vi "SJ_old_results plotter.vi"() -> ()   [LabVIEW 2022 SP3]
uses:
  Controls/Inst_type.ctl
  Controls/Instrument_Array.ctl
  Controls/Analysis_info_cluster.ctl
  Controls/SJ_Test_Matrix.ctl
  <vilib>/Analysis/NI_AALBase.lvlib
  <vilib>/Analysis/1siggen.llb/Ramp Pattern by Samples.vi
  <vilib>/Analysis/baseanly.llb/Scale 1D.vi
  <vilib>/Analysis/NI_AALPro.lvlib
  <vilib>/Analysis/baseanly.llb/Scale 2D.vi
  <vilib>/gmath/NumericalOptimization/stopping criteria.ctl
  <vilib>/gmath/NI_Gmath.lvlib
panel:
  out "size(s)":i32[](array[numeric])
  out "Tab Control":enum32{"Animate", "Parabola"}(tab)
  out "Displacement Graph":cluster{"Y=(X-offset)/scale":dbl[], dbl[]}[](graph)
  out "Progress...":sgl(slide) scale=0.0..1.0
  out "Error":cluster{dbl[], dbl[]}[](graph)
  out "Phi":cluster{dbl[], dbl[]}[](graph)
  out "Beta":cluster{dbl[], dbl[]}[](graph)
  in  "stopping criteria":T1={"function tolerance"=0.001, "parameter tolerance"=0.001, "max iterations"=100, "max function calls"=1000, "gradient tolerance"=0.001, "max time (sec)"=-1.0}
  in  "Fit Parabola":bool
  in  "Load data":bool
  in  "Raw Data Folder":path=path "F:/Enflo_Data_Local/2011/Aero_Tunnel/nick_martin/Raw_Measurements/11-2011/New_SJ_TestI_xls"
  in  "Play Button":bool
  out "Message":string
  in  "Frequencies":i32[](listbox)
  in  "Amplitudes":i32[](listbox)
  in  "Stop Button":bool
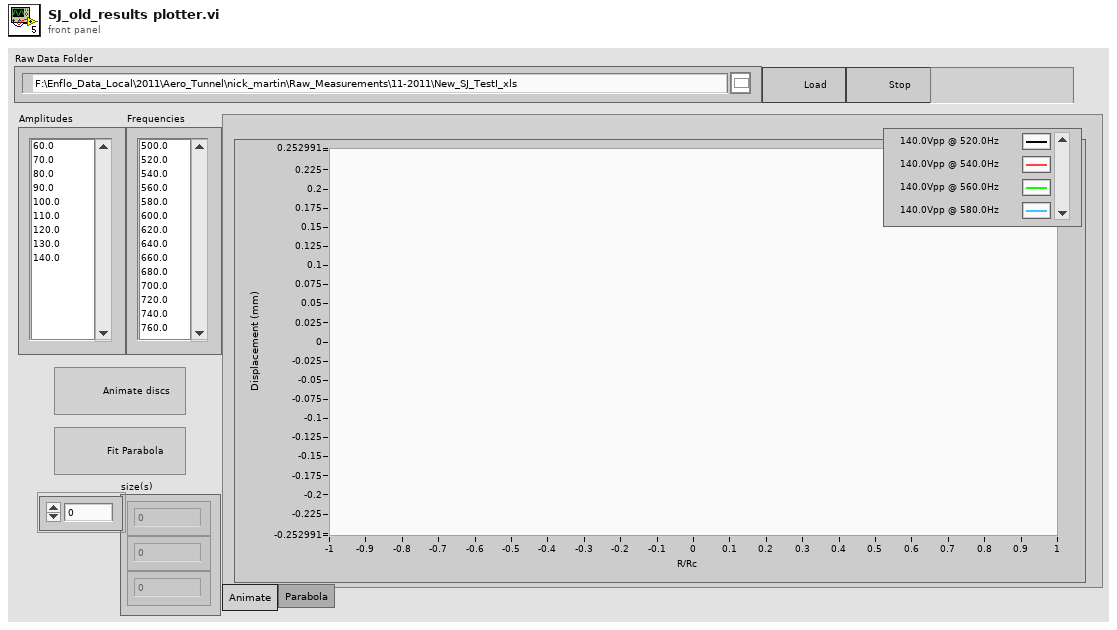
[diagram p1: front panel]
types:
  T1 = typedef "NI_Gmath.lvlib/stopping criteria.ctl" = cluster{"function tolerance":dbl, "parameter tolerance":dbl, "max iterations":i32, "max function calls":i32, "gradient tolerance":dbl, "max time (sec)":dbl}
  T2 = typedef "SJ_Test_Matrix.ctl" = cluster{"Channel Data":cluster{"Amplitude (V)":dbl, "Phase Average":dbl[][], "Phase Angle":dbl[], "Frequency (Hz)":dbl, "AS Freq":dbl, "Zero":dbl, "Analysis info cluster":T3, "Radius":dbl[], "||beta||":dbl, "Phi":dbl, "||xd'||":dbl, "xd":dbl[], "||xd||":dbl, "xd'":dbl[], "beta":dbl[]}[]}
  T3 = typedef "Analysis_info_cluster.ctl" = cluster{"Colour":u32, "Inst type":T4, "Inst name":string, "Symbol":string, "Code name":string, "Extra Info":string, "Inst Array":T5, "Extra Titles":string[], "Extra Values":string[], "U":dbl, "u^2":dbl, "u^3":dbl, "u^4":dbl, "Skew_u":dbl, "Kurt_u":dbl, "Sd Error in Mean":dbl, "% u'/U":dbl, "X":dbl, "Y":dbl, "Z":dbl, "Timescale integral Estimate":dbl, "Sd Error in Variance":dbl, "Calib File":path, "Calib Constants":dbl[], "Output Position":bool, "Stats":enum16{"None", "Basic", "Full"}, "Av Sampling Rate":dbl, "Av No of Samples":dbl, "Total Meas Time (s)":dbl, "ADAM Ch Name":string, "Max value":dbl, "Min value":dbl, "Req Sample Rate Hz":dbl, "Sync Delay Time (s)":dbl, "Ch No":i16, "Device":string, "Use Latest Calib":bool, "Port":string, "Metadata Ch Names":string[], "Metadata Ch Values":string[], "Label":string}
  T4 = typedef "Inst_type.ctl" = enum16{"Raw voltage", "Raw with zero offsetting", "Propeller anemometer", "Pressure Transducer", "Pitot-static tube", "Hot wire", "Cross wire 1", "Cross wire 2", "Generic Linear", "Generic Polynomial", "Generic BackPoly", "Fast FID", "Thermocouple", "Cold wire", "Pulsed Wire", "LDA Vel", "LDA Tran time", "LDA Arr time", "Microphone"}
  T5 = typedef "Instrument_Array.ctl" = enum16{"PWA", "LDA", "Analogue"}
  T6 = cluster{"Amplitude (V)":dbl, "Phase Average":dbl[][], "Phase Angle":dbl[], "Frequency (Hz)":dbl, "AS Freq":dbl, "Zero":dbl, "Analysis info cluster":T3, "Radius":dbl[], "||beta||":dbl, "Phi":dbl, "||xd'||":dbl, "xd":dbl[], "||xd||":dbl, "xd'":dbl[], "beta":dbl[]}[]
  T7 = cluster{"Amplitude (V)":dbl, "Phase Average":dbl[][], "Phase Angle":dbl[], "Frequency (Hz)":dbl, "AS Freq":dbl, "Zero":dbl, "Analysis info cluster":T3, "Radius":dbl[], "||beta||":dbl, "Phi":dbl, "||xd'||":dbl, "xd":dbl[], "||xd||":dbl, "xd'":dbl[], "beta":dbl[]}
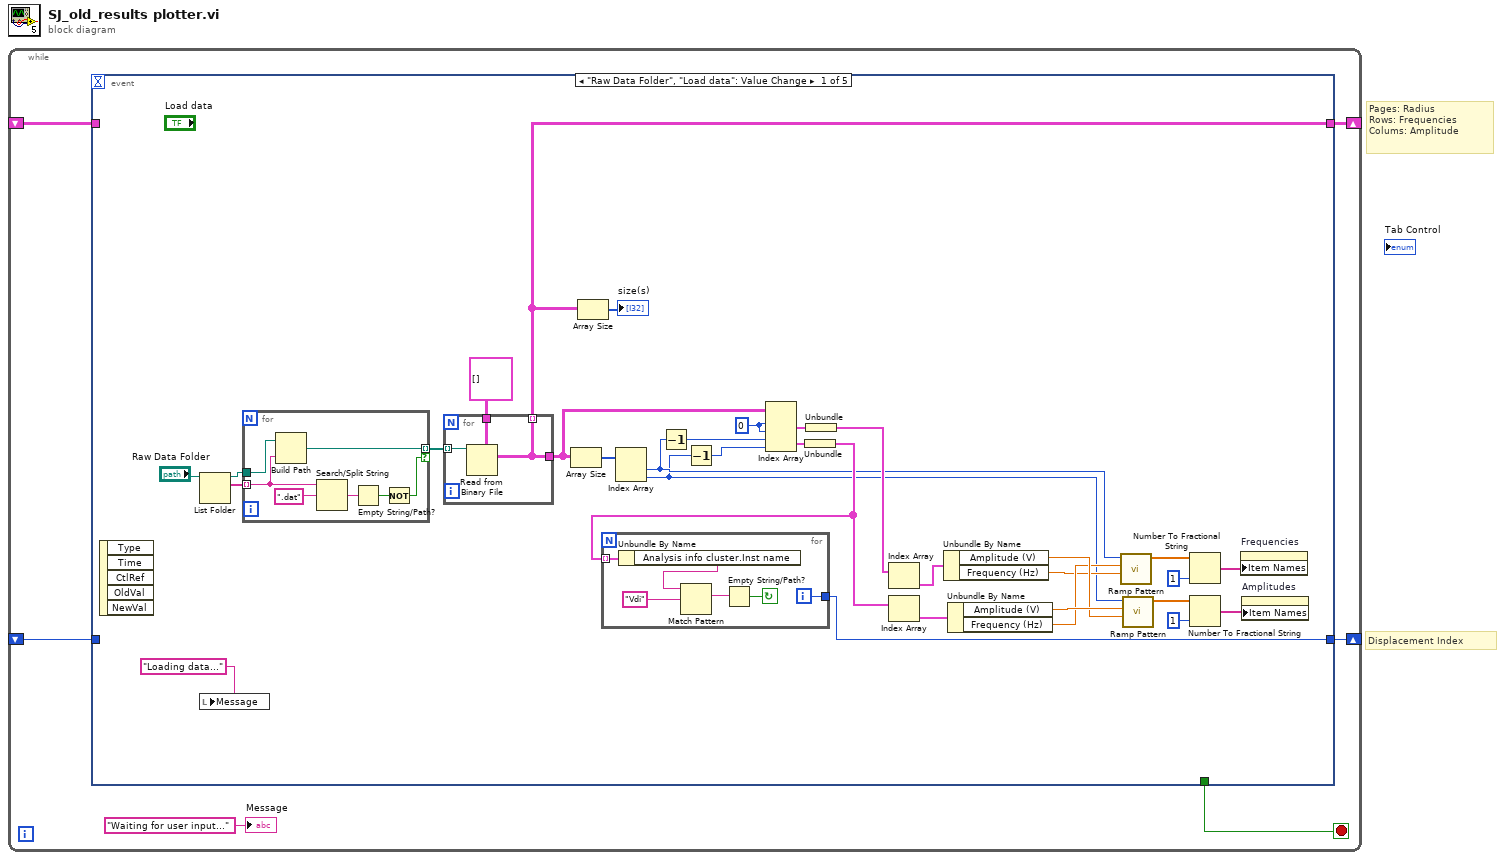
[diagram p0: block diagram]
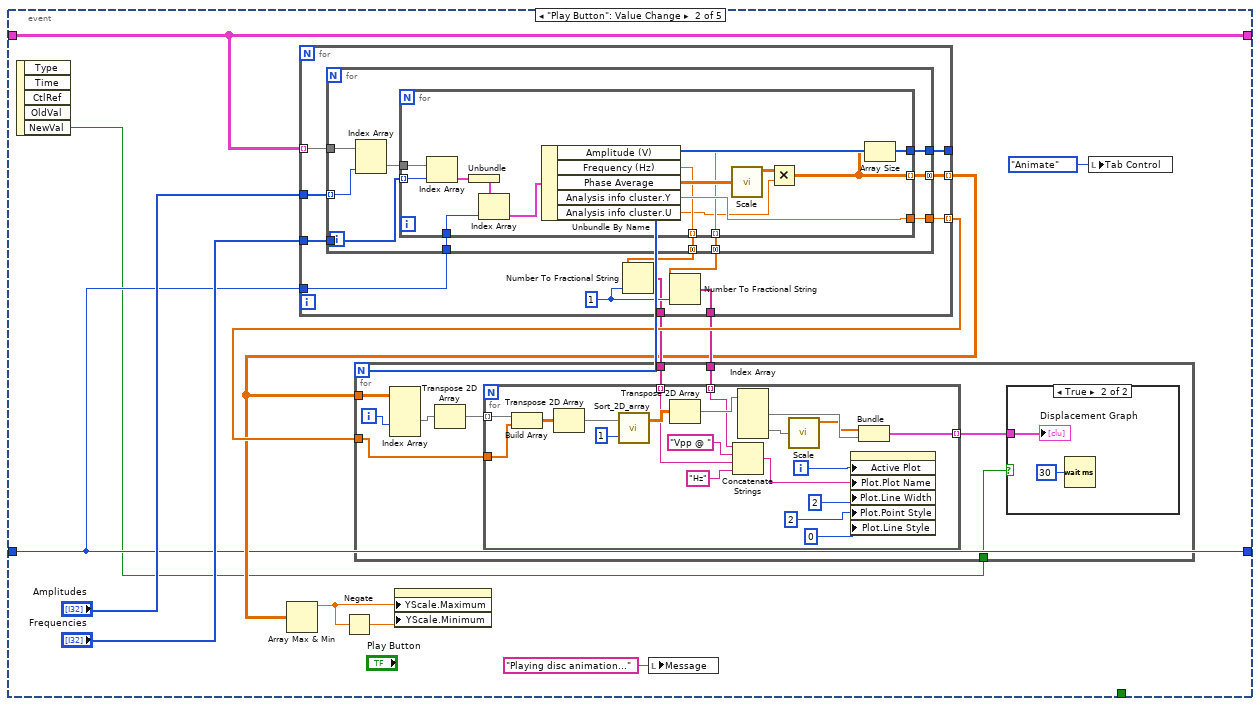
[diagram p2: hidden frame]
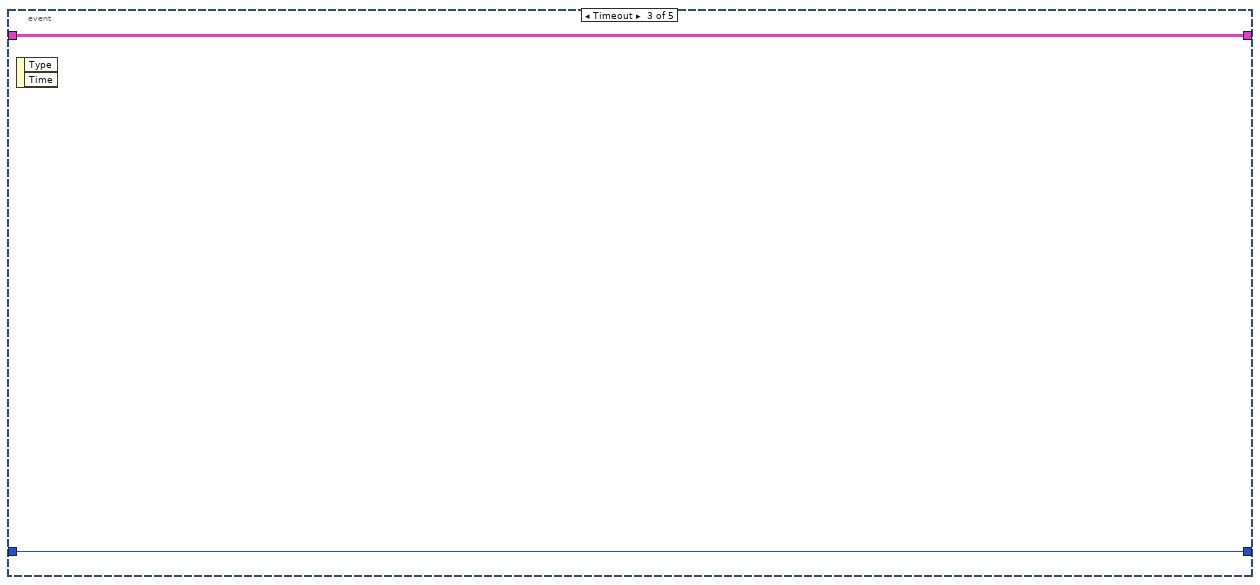
[diagram p4: hidden frame]
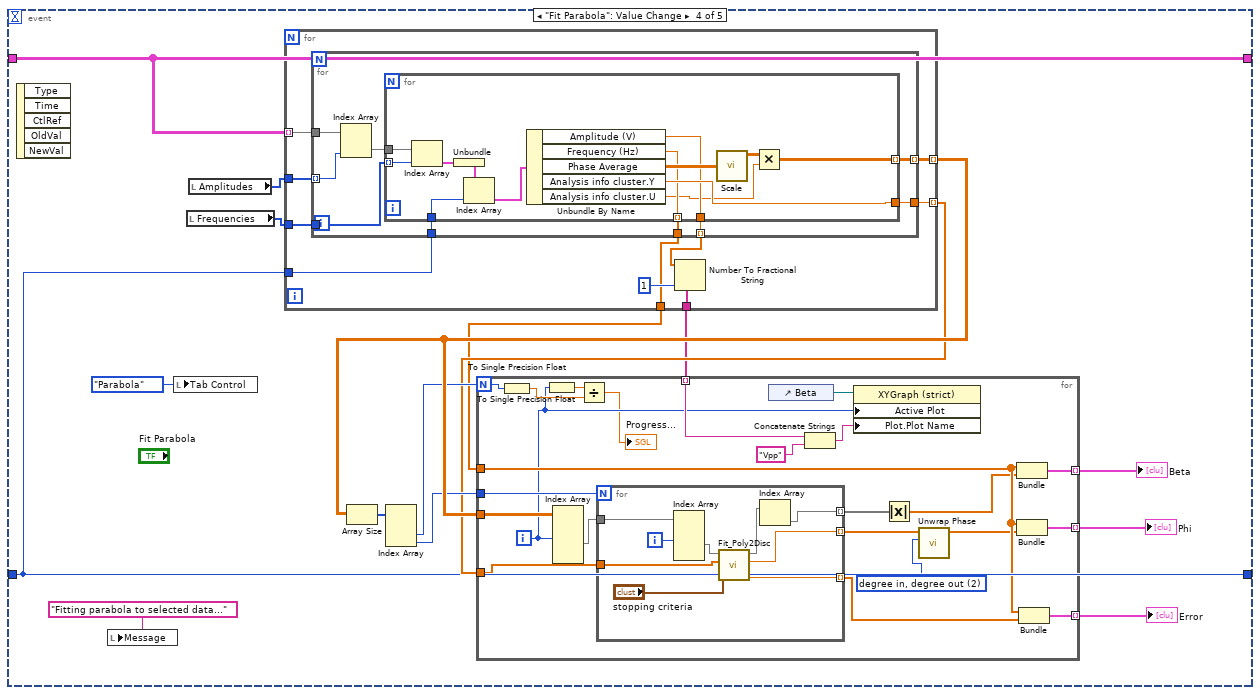
[diagram p5: hidden frame]
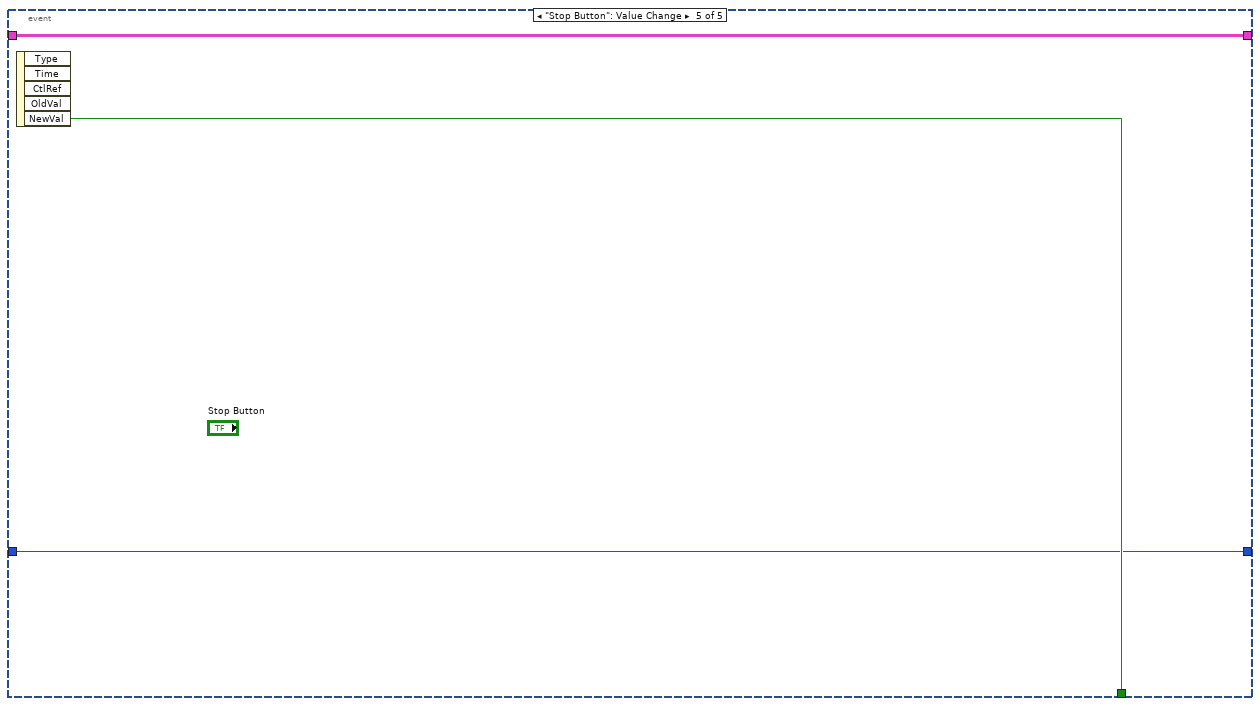
[diagram p6: hidden frame]
diagram:
  # "Displacement Index"
  # "Pages: Radius\nRows: Frequencies\nColums: Amplitude"
  n1 = while {
    shift-right: [w2] -> _
    shift-left: _ -> [w5]
    shift-right: [w3] -> _
    shift-left: _ -> [w4]
    stop <- w6 stop-if-true
    n2 = event shown="[0] \"Raw Data Folder\", \"Load data\": Value Change" {
      selector: _ -> [_ _ _ _ _]
      dyn-events: _ -> [_ _ _ _ _]
      timeout: _ -> [_ _ _ _ _]
      tunnel: [_ _ _ _ w220] -> w6
      tunnel: w5 -> [_ w65 w136 w138 w219]
      tunnel: w4 -> [_ w57 w137 w142 w218]
      tunnel: [w10 w57 w137 w142 w218] -> w3
      tunnel: [w8 w65 w136 w138 w219] -> w2
      event "Raw Data Folder", "Load data": Value Change {
        w17 = 0 ("index (row)")
        n3 = event-data() -> ()  [unwired: 1 in, 5 out]
        n4 = List Folder(path="Raw Data Folder") -> (path out=w36:path, filenames=w37:string[])  [unwired: 3 in, 2 out]
        n5 = local write "Message"("Loading data..." ("Message")) -> ()
        n6 = for {
          tunnel: w37 -> [w49] mode=indexing
          tunnel: [w48] -> w23 mode=indexing if=w52
          tunnel: w36 -> [w50]
          n7 = Build Path(base path=w50, name or relative path=w49) -> (appended path=w48:path)
          n8 = Search/Split String(string=w49, search string/char (-)=".dat" ("regular expression")) -> (match + rest of string=w51:string)  [unwired: 1 in, 2 out]
          n9 = Empty String/Path?(string/path=w51) -> (empty?=w53:bool)
          n10 = Not(x=w53) -> (.not. x?=w52:bool)
        }
        n11 = for {
          tunnel: w23 -> [w47] mode=indexing
          tunnel: T2[][] [] -> [w46]
          tunnel: [w45] -> w15
          tunnel: [w45] -> w8 mode=indexing
          n12 = Read from Binary File(5:w46, 11:w47) -> (2:w45:T2[][])  [unwired: 4 in, 3 out]
        }
        n13 = Array Size(array=w15) -> (size(s)=w16:i32[])
        n14 = Array Size(array=w8) -> (size(s)=→"size(s)":i32[])
        n15 = Index Array(array=w16) -> (element #1=w12:i32, element #2=w11:i32)  [unwired: 2 in]
        n16 = Decrement(x=w12) -> (x-1=w18:i32)
        n17 = Decrement(x=w11) -> (x-1=w19:i32)
        n18 = Index Array(array=w15, index (row) #1=w17, index (col) #1=w17, index (row) #2=w18, index (col) #2=w19) -> (element #1=w20:T2, element #2=w21:T2)
        n19 = Unbundle(w21) -> ("Channel Data"=w14:T6)
        n20 = for {
          tunnel: w14 -> [w44] mode=indexing
          tunnel: [w39] -> w10
          i -> [w39]
          stop <- w40 continue-if-true
          n21 = Unbundle By Name(w44) -> ("Analysis info cluster.Inst name"=w43:string)
          n22 = Match Pattern(string=w43, regular expression="Vdi") -> (match substring=w41:string)  [unwired: 1 in, 3 out]
          n23 = Empty String/Path?(string/path=w41) -> (empty?=w40:bool)
        }
        n24 = Unbundle(w20) -> ("Channel Data"=w13:T6)
        n25 = Index Array(array=w13) -> (element=w31:T7)  [unwired: 1 in]
        n26 = Index Array(array=w14) -> (element=w32:T7)  [unwired: 1 in]
        n27 = Unbundle By Name(w31) -> ("Amplitude (V)"=w34:dbl, "Frequency (Hz)"=w30:dbl)
        n28 = Unbundle By Name(w32) -> ("Amplitude (V)"=w35:dbl, "Frequency (Hz)"=w33:dbl)
        n29 = call-poly <vilib>:"Ramp Pattern.vi"("start"=w30, "end"=w33, "samples"=w12) -> ("Ramp Pattern"=w29:dbl[])  [unwired: 7 in, 1 out]
        n30 = call-poly <vilib>:"Ramp Pattern.vi"("start"=w34, "end"=w35, "samples"=w11) -> ("Ramp Pattern"=w27:dbl[])  [unwired: 7 in, 1 out]
        n31 = Number To Fractional String(number=w29, precision (6)=i16 1) -> (F-format string=w28:string[])  [unwired: 2 in]
        n32 = Number To Fractional String(number=w27, precision (6)=i16 1) -> (F-format string=w26:string[])  [unwired: 2 in]
        n33 = property on="Frequencies" class="LstBox (strict)"("Item Names"=w28) -> ()  [unwired: 2 in, 2 out]
        n34 = property on="Amplitudes" class="LstBox (strict)"("Item Names"=w26) -> ()  [unwired: 2 in, 2 out]
      }
      event "Play Button": Value Change {
        n35 = event-data() -> ("NewVal"=w56:bool)  [unwired: 1 in, 4 out]
        n36 = for {
          tunnel: w65 -> [w111] mode=indexing
          tunnel: [w110] -> w66 mode=indexing
          tunnel: "Amplitudes" -> [w109]
          tunnel: "Frequencies" -> [w108]
          tunnel: [w107] -> w60 mode=indexing
          tunnel: [w106] -> w67
          tunnel: [w104] -> w64
          tunnel: [w101] -> w63
          tunnel: w57 -> [w100]
          w102 = i16 1 ("precision (6)")
          n37 = for {
            tunnel: w111 -> [w121]
            tunnel: [w119] -> w110
            tunnel: [w118] -> w107 mode=concatenating
            tunnel: w109 -> [w117] mode=indexing
            tunnel: w108 -> [w116]
            tunnel: [w115] -> w106
            tunnel: [w114] -> w103 mode=concatenating
            tunnel: [w113] -> w105 mode=concatenating
            tunnel: w100 -> [w112]
            n38 = Index Array(array=w121, index (col)=w117) -> (element=w120:T2[])  [unwired: 1 in]
            n39 = for {
              tunnel: w120 -> [w135]
              tunnel: [w131] -> w119
              tunnel: [w123] -> w118 mode=indexing
              tunnel: w116 -> [w128] mode=indexing
              tunnel: [w127] -> w115
              tunnel: [w126] -> w114 mode=indexing
              tunnel: [w125] -> w113 mode=indexing
              tunnel: w112 -> [w122]
              n40 = Index Array(array=w135, index=w128) -> (element=w134:T2)
              n41 = Unbundle(w134) -> ("Channel Data"=w133:T6)
              n42 = Index Array(array=w133, index=w122) -> (element=w132:T7)
              n43 = Unbundle By Name(w132) -> ("Amplitude (V)"=w125:dbl, "Frequency (Hz)"=w126:dbl, "Phase Average"=w130:dbl[][], "Analysis info cluster.Y"=w131:dbl, "Analysis info cluster.U"=w124:dbl)
              n44 = call-poly <vilib>:"Scale.vi"("X"=w130) -> ("Y=(X-offset)/scale"=w129:dbl[][])  [unwired: 3 out]
              n45 = Multiply(x=w129, y=w124) -> (x*y=w123:dbl[][])
              n46 = Array Size(array=w123) -> (size(s)=w127:i32[])
            }
          }
          n47 = Number To Fractional String(number=w103, precision (6)=w102) -> (F-format string=w101:string[])  [unwired: 2 in]
          n48 = Number To Fractional String(number=w105, precision (6)=w102) -> (F-format string=w104:string[])  [unwired: 2 in]
        }
        n49 = Array Max & Min(array=w60) -> (max value=w62:dbl)  [unwired: 3 out]
        n50 = Negate(x=w62) -> (-x=w61:dbl)
        n51 = for {
          N: w67 -> [_]
          tunnel: w66 -> [w77]
          tunnel: w60 -> [w72]
          tunnel: w56 -> [w75]
          tunnel: w64 -> [w74]
          tunnel: w63 -> [w73]
          i -> [w69]
          n52 = Index Array(array=w72, index (dim 2)=w69) -> (element=w70:dbl[][][])  [unwired: 3 in]
          n53 = Transpose 2D Array(2D array=w70) -> (transposed array=w71:dbl[][])
          n54 = for {
            tunnel: w71 -> [w99] mode=indexing
            tunnel: w77 -> [w87]
            tunnel: [w84] -> w76 mode=indexing
            tunnel: w74 -> [w92] mode=indexing
            tunnel: w73 -> [w90] mode=indexing
            i -> [w82]
            n55 = Build Array(w99, w87) -> (w98:dbl[][])
            n56 = Transpose 2D Array(2D array=w98) -> (transposed array=w94:dbl[][])
            n57 = call "Sort_2D_array.vi"("Column index to sort on"=1, "unsorted array"=w94) -> ("sorted array"=w96:dbl[][])  [unwired: 1 out]
            n58 = Transpose 2D Array(2D array=w96) -> (transposed array=w93:dbl[][])
            n59 = Concatenate Strings(w92, "Vpp @ " ("string"), w90, "Hz" ("string")) -> (w88:string)
            n60 = Index Array(array=w93) -> (element #1=w95:dbl[], element #2=w86:dbl[])  [unwired: 4 in]
            n61 = call-poly <vilib>:"Scale.vi"("X"=w86) -> ("Y=(X-offset)/scale"=w85:dbl[])  [unwired: 3 out]
            n62 = property on="Displacement Graph" class="XYGraph (strict)"("Active Plot"=w82, "Plot.Plot Name"=w88, "Plot.Line Width"=u8 2, "Plot.Point Style"=u8 2, "Plot.Line Style"=u8 0) -> ()  [unwired: 2 in, 2 out]
            n63 = Bundle("Y=(X-offset)/scale"=w85, w95) -> (w84:cluster{"Y=(X-offset)/scale":dbl[], dbl[]})  [unwired: 1 in]
          }
          n64 = case shown="True" w75 {
            tunnel: w76 -> [_ w78]
            frame False {
            }
            frame True {
              n65 = Wait (ms)(milliseconds to wait=u32 30) -> ()  [unwired: 1 out]
              "Displacement Graph" <- w78
            }
          }
        }
        n66 = property on="Displacement Graph" class="XYGraph (strict)"("YScale.Maximum"=w62, "YScale.Minimum"=w61) -> ()  [unwired: 2 in, 2 out]
        n67 = local write "Message"("Playing disc animation..." ("Message")) -> ()
        n68 = local write "Tab Control"(enum32{"Animate", "Parabola"}."Animate" ("Tab Control")) -> ()
      }
      event Timeout {
        n69 = event-data() -> ()  [unwired: 1 in, 2 out]
      }
      event "Fit Parabola": Value Change {
        n70 = event-data() -> ()  [unwired: 1 in, 5 out]
        n71 = local write "Message"("Fitting parabola to selected data..." ("Message")) -> ()
        n72 = local write "Tab Control"(enum32{"Animate", "Parabola"}."Parabola" ("Tab Control")) -> ()
        n73 = local read "Frequencies"() -> (w143:i32[])
        n74 = local read "Amplitudes"() -> (w144:i32[])
        n75 = for {
          tunnel: w138 -> [w195] mode=indexing
          tunnel: [w194] -> w148 mode=indexing
          tunnel: w144 -> [w193]
          tunnel: w143 -> [w192]
          tunnel: [w191] -> w152 mode=indexing
          tunnel: [w190] -> w145
          tunnel: w142 -> [w188]
          tunnel: [w186] -> w147
          n76 = for {
            tunnel: w195 -> [w204]
            tunnel: [w202] -> w194
            tunnel: [w201] -> w191 mode=indexing
            tunnel: w193 -> [w200] mode=indexing
            tunnel: w192 -> [w199]
            tunnel: [w198] -> w186
            tunnel: [w197] -> w187 mode=indexing
            tunnel: w188 -> [w196]
            n77 = Index Array(array=w204, index (col)=w200) -> (element=w203:T2[])  [unwired: 1 in]
            n78 = for {
              tunnel: w203 -> [w217]
              tunnel: [w213] -> w202
              tunnel: [w206] -> w201 mode=indexing
              tunnel: w199 -> [w210] mode=indexing
              tunnel: [w209] -> w198 mode=indexing
              tunnel: [w208] -> w197
              tunnel: w196 -> [w205]
              n79 = Index Array(array=w217, index=w210) -> (element=w216:T2)
              n80 = Unbundle(w216) -> ("Channel Data"=w215:T6)
              n81 = Index Array(array=w215, index=w205) -> (element=w214:T7)
              n82 = Unbundle By Name(w214) -> ("Amplitude (V)"=w208:dbl, "Frequency (Hz)"=w209:dbl, "Phase Average"=w212:dbl[][], "Analysis info cluster.Y"=w213:dbl, "Analysis info cluster.U"=w207:dbl)
              n83 = call-poly <vilib>:"Scale.vi"("X"=w212) -> ("Y=(X-offset)/scale"=w211:dbl[][])  [unwired: 3 out]
              n84 = Multiply(x=w211, y=w207) -> (x*y=w206:dbl[][])
            }
          }
          n85 = Number To Fractional String(number=w187, precision (6)=i16 1) -> (F-format string=w190:string[])  [unwired: 2 in]
        }
        n86 = Array Size(array=w152) -> (size(s)=w151:i32[])
        n87 = Index Array(array=w151) -> (element #2=w150:i32, element #3=w149:i32)  [unwired: 3 in, 1 out]
        n88 = for {
          N: w150 -> [w161]
          tunnel: w152 -> [w176]
          tunnel: w149 -> [w174]
          tunnel: w148 -> [w173]
          tunnel: w147 -> [w166]
          tunnel: [w169] -> w146 mode=indexing
          tunnel: [w168] -> w140 mode=indexing
          tunnel: [w167] -> w139 mode=indexing
          tunnel: w145 -> [w165] mode=indexing
          i -> [w158]
          w154 = 2 items=["radian in, radian out", "radian in, degree out", "degree in, degree out", "degree in, radian out"] ("phase unit")
          n89 = To Single Precision Float(number=w161) -> (single precision float=w160:sgl)
          n90 = To Single Precision Float(number=w158) -> (single precision float=w159:sgl)
          n91 = Index Array(array=w176, index (dim 1)=w158) -> (element=w175:dbl[][][][])  [unwired: 4 in]
          n92 = Divide(x=w159, y=w160) -> (x/y=→"Progress...":sgl)
          n93 = for {
            N: w174 -> [_]
            tunnel: w175 -> [w185]
            tunnel: w173 -> [w183]
            tunnel: [w181] -> w172 mode=indexing
            tunnel: [w180] -> w171 mode=indexing
            tunnel: [w179] -> w170 mode=indexing
            i -> [w184]
            n94 = Index Array(array=w185, index (dim 1)=w184) -> (element=w178:dbl[][][])  [unwired: 3 in]
            n95 = call "Fit_Poly2Disc.vi"("stopping criteria"="stopping criteria", "Rc"=w183, "Xd(t,r)"=w178) -> ("f(minimum)"=w179:dbl, "Sine Phase"=w180:dbl, 3:w182)  [unwired: 5 in, 1 out]
            n96 = Index Array(array=w182) -> (element=w181)  [unwired: 1 in]
          }
          n97 = control-ref of="Beta"() -> (w164:refnum<vi>)
          n98 = Concatenate Strings(w165, "Vpp" ("string")) -> (w163:string)
          n99 = property class="XYGraph (strict)"(reference=w164, "Active Plot"=w158, "Plot.Plot Name"=w163) -> ()  [unwired: 1 in, 2 out]
          n100 = Absolute Value(x=w172) -> (abs(x)=w156:dbl[])
          n101 = call <vilib>:"Unwrap Phase.vi"("phase unit"=w154, "Phase"=w171) -> ("Unwrapped Phase"=w155:dbl[])  [unwired: 8 in, 1 out]
          n102 = Bundle(w166, w156) -> (w169:cluster{dbl[], dbl[]})  [unwired: 1 in]
          n103 = Bundle(w166, "Unwrapped Phase"=w155) -> (w168:cluster{dbl[], "Unwrapped Phase":dbl[]})  [unwired: 1 in]
          n104 = Bundle(w166, w170) -> (w167:cluster{dbl[], dbl[]})  [unwired: 1 in]
        }
        "Beta" <- w146
        "Phi" <- w140
        "Error" <- w139
      }
      event "Stop Button": Value Change {
        n105 = event-data() -> ("NewVal"=w220:bool)  [unwired: 1 in, 4 out]
      }
    }
    "Message" <- "Waiting for user input..." ("Message")
  }
